vi "mks946_get_all.vi"(6 "err_in":errorcluster, 7 "mks946_visa":refnum<visa-resource-name>="COM3", 10 "mks946_ch":dbl=1.0, 11 "mks946_id":i32=253) -> (0 "mks946_st":bool=TRUE, 3 "mks946_res":T1={"res_ch"=enum."1", "res_val"=743.4, "res_id"=253, "res_msg"="OK"})   [LabVIEW 2019]
uses:
  ctrl_mks946_res.ctl
panel:
  in  "mks946_comm 2":string="FR"
  out "mks946_res 2":T1={"res_ch"=enum."3", "res_val"=-3.6, "res_id"=253, "res_msg"="OK"}
  out "mks946_st 2":bool=TRUE
  in  "mks946_ch 2":dbl=3.0
  out "err_out 2":errorcluster={"status"=FALSE, "code"=1073676294, "source"="VISA Read in mks946_sub_get.vi->mks946_get_all.vi"}
  in  "mks946_comm":string="PR"
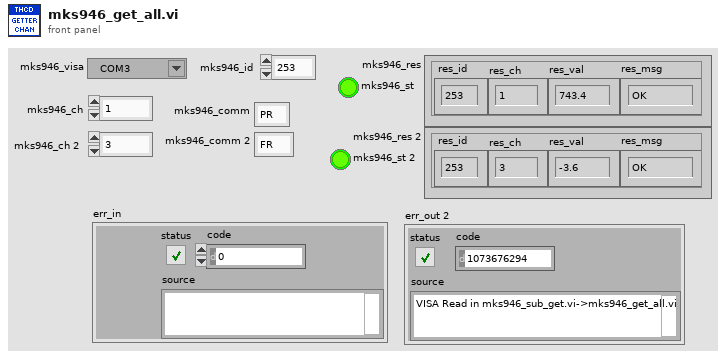
[diagram p1: front panel]
types:
  T1 = typedef "ctrl_mks946_res.ctl" = cluster{"res_ch":enum8{"ERR", "1", "2", "3", "4", "5", "6"}, "res_val":dbl, "res_id":u8, "res_msg":string}
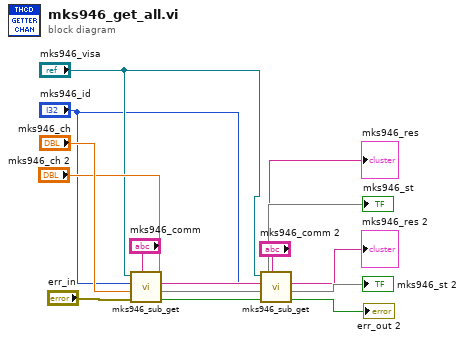
[diagram p0: block diagram]
diagram:
  n1 = call "mks946_sub_get.vi"("VISA_ref_in"="mks946_comm", 8:"err_in", 9:"mks946_ch", "command"="mks946_id", "address"="mks946_visa") -> ("status"=w3:bool, 1:→"mks946_st", "message"=→"mks946_res":string)  [unwired: 1 in, 3 out]
  n2 = call "mks946_sub_get.vi"("VISA_ref_in"="mks946_comm 2", 8:w3, 9:"mks946_ch 2", "command"="mks946_id", "address"="mks946_visa") -> ("status"=→"err_out 2":bool, 1:→"mks946_st 2", "message"=→"mks946_res 2":string)  [unwired: 1 in, 3 out]
